vi "Teleop.vi"(10 "Match Info":T4={"Autonomous Elapsed Seconds"=0.0, "TeleOp Elapsed Seconds"=0.0, "Disabled Elapsed Seconds"=0.0, "Visited Autonomous"=FALSE, "Visited TeleOp"=FALSE, "Visited Disabled"=FALSE, "Autonomous Settings"={"Autonomous Style"=enum."Independent", "VI Refnum"=refnum}}, 11 "Call Context":T5) -> ()   [LabVIEW 2016]
doc: "This VI is called for each TeleOp packet received from the DS where the robot is not disabled. It is often used to read from the joysticks and update I/O or to update setpoints for timed control loops. It should complete and return within 20 milliseconds or it may miss DS packets."
uses:
  <vilib>/Rock Robotics/WPI/DriverStation/WPI_DriverStationDerivedRobotMode.ctl
  <vilib>/Rock Robotics/WPI/DriverStation/WPI_DriverStationMatch Info.ctl
  <vilib>/Rock Robotics/WPI/PWM/Servo/WPI_ServoDeviceRef.ctl
  <vilib>/Rock Robotics/SystemInterfaces/DIO/FPGA_DIOPWMChannel.ctl
  <vilib>/Rock Robotics/WPI/PWM/WPI_PWMDeadband.ctl
  <vilib>/Rock Robotics/WPI/Utilities/WPI_GetSetVariantRefNum.vi
  <vilib>/Rock Robotics/Network Tables/NT Write Boolean Array.vi
  <vilib>/Rock Robotics/Network Tables/NT Write Numeric Array.vi
  <vilib>/Rock Robotics/Network Tables/NT Read Boolean.vi
  <vilib>/Rock Robotics/Network Tables/NT Read Number.vi
  <vilib>/Rock Robotics/WPI/RobotDrive/WPI_RobotDriveArcadeDrive_Standard(NoSaturation).vi
  <vilib>/Rock Robotics/WPI/Power/WPI_Power Get 6Volt Rail Voltage and Current.vi
panel:
  in  "x 2":dbl=0.2 format="%#_13g"
  in  "x":dbl=0.2 format="%#_13g"
  out "all currents (A)":dbl[](array[numeric])
  out "current (A)":dbl
  out "all currents (A) 2":dbl[](array[numeric])
  out "PDP current (A)":dbl
  out "PDP voltage (V)":dbl
  out "Power (W)":dbl
  out "Energy (J)":dbl
  out "6 volt rail current (A)":dbl
  out "6 volt rail voltage (V)":dbl
  out "5V User Rail Brown Out":bool
  out "6 V User Rail Short":bool
  out "5 V User Rail Short":bool
  out "3.3V User Rail Short":bool
  out "Input Voltage Brown Out":bool
  out "roboRIO input current (A)":dbl
  out "roboRIO input voltage (V)":dbl
  out "Encoder Status":string
  out "Encoder Rate":dbl
  out "Encoder Direction":string
  out "Encoder Distance":dbl
  out "Gripper Position":dbl
  out "Gripper Servo Device Ref":T1={"DeviceStatus"={"status"=FALSE, "code"=0, "source"=""}, "PWM Channel"=enum."Invalid", "DeadBand"={"Name"="", "maxPositivePwm"=0, "minPositivePwm"=0, "centerPwm"=0, "maxNegativePwm"=0, "minNegativePwm"=0, "angularRange"=0}}
  out "Arm Position":dbl
  out "Arm Servo Device Ref":T1={"DeviceStatus"={"status"=FALSE, "code"=0, "source"=""}, "PWM Channel"=enum."Invalid", "DeadBand"={"Name"="", "maxPositivePwm"=0, "minPositivePwm"=0, "centerPwm"=0, "maxNegativePwm"=0, "minNegativePwm"=0, "angularRange"=0}}
  in  "Gripper Scale Factor":dbl=0.004
  in  "Arm Scale Factor":dbl=0.004
  out "Sample Slider 0":dbl(slide) scale=0.0..5.0
  out "Sample Boolean 1":bool
  out "Sample Boolean 0":bool
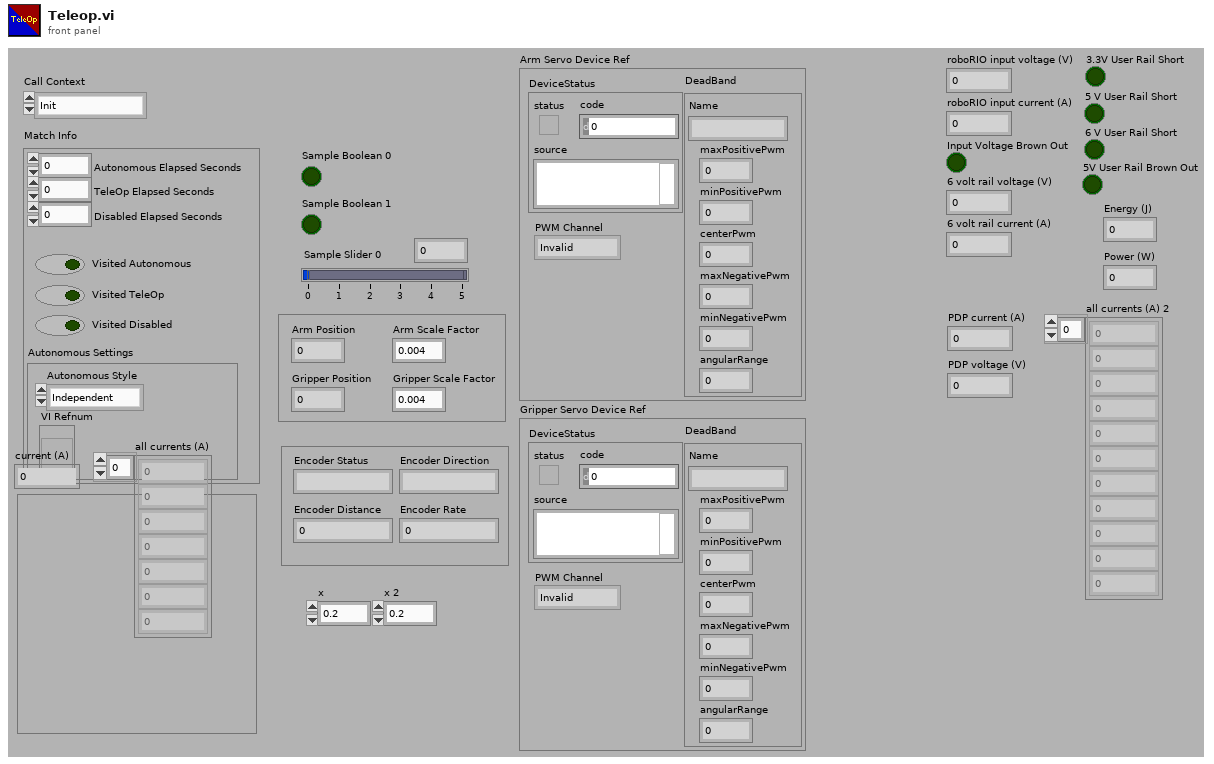
[diagram p1: front panel]
types:
  T1 = typedef "WPI_ServoDeviceRef.ctl" = cluster{"DeviceStatus":errorcluster, "PWM Channel":T2, "DeadBand":T3}
  T2 = typedef "FPGA_DIOPWMChannel.ctl" = enum8{"PWM 0", "PWM 1", "PWM 2", "PWM 3", "PWM 4", "PWM 5", "PWM 6", "PWM 7", "PWM 8", "PWM 9", "PWM MXP 0", "PWM MXP 1", "PWM MXP 2", "PWM MXP 3", "PWM MXP 4", "PWM MXP 5", "PWM MXP 6", "PWM MXP 7", "PWM MXP 8", "PWM MXP 9", "Invalid"}
  T3 = typedef "WPI_PWMDeadband.ctl" = cluster{"Name":string, "maxPositivePwm":i32, "minPositivePwm":i32, "centerPwm":i32, "maxNegativePwm":i32, "minNegativePwm":i32, "angularRange":u16}
  T4 = typedef "WPI_DriverStationMatch Info.ctl" = cluster{"Autonomous Elapsed Seconds":dbl, "TeleOp Elapsed Seconds":dbl, "Disabled Elapsed Seconds":dbl, "Visited Autonomous":bool, "Visited TeleOp":bool, "Visited Disabled":bool, "Autonomous Settings":cluster{"Autonomous Style":enum16{"Iterative", "Independent"}, "VI Refnum":refnum<vi>}}
  T5 = typedef "WPI_DriverStationDerivedRobotMode.ctl" = enum16{"Init", "Execute", "Stop"}
  T6 = typedef "WPI_EncoderDevRef.ctl" = cluster{"DevStatus":errorcluster, "EncoderIndex":T7, "CounterIndex":T8, "DistancePerCount":dbl, "Decoding Type":T9}
  T7 = typedef "FPGA_EncoderIdx.ctl" = enum8{"Enc 0", "Enc 1", "Enc 2", "Enc 3", "Enc 4", "Enc 5", "Enc 6", "Enc 7", "Invalid"}
  T8 = typedef "FPGA_CounterCtrSystemIndex.ctl" = enum8{"Ctr 0", "Ctr 1", "Ctr 2", "Ctr 3", "Ctr 4", "Ctr 5", "Ctr 6", "Ctr 7", "Invalid"}
  T9 = typedef "WPI_EncoderType.ctl" = enum16{"1x", "2x", "4x"}
  T10 = typedef "WPI_RobotDriveDevRef.ctl" = cluster{"DevStatus":errorcluster, "Motors[]":T11[], "Square Inputs":bool, "Max Output":dbl}
  T11 = typedef "WPI_MotorControlDeviceRef.ctl" = cluster{"DeviceStatus":errorcluster, "Type":T12, "PWM":cluster{"PWM Channel":T2, "DeadBand":T3}, "CAN":cluster{"Device Number":u8, "SetOutput VI Ref":variant, "GetOutput VI Ref":variant, "Enable VI Ref":variant, "Disable VI Ref":variant, "Data":variant}, "Invert":bool}
  T12 = typedef "WPI_MotorControlType.ctl" = enum16{"PWM", "CAN"}
  T13 = typedef "WPI_JoystickDevRef.ctl" = cluster{"Device":T14}
  T14 = typedef "WPI_JoystickDeviceEnum.ctl" = enum16{"USB 0", "USB 1", "USB 2", "USB 3", "USB 4", "USB 5"}
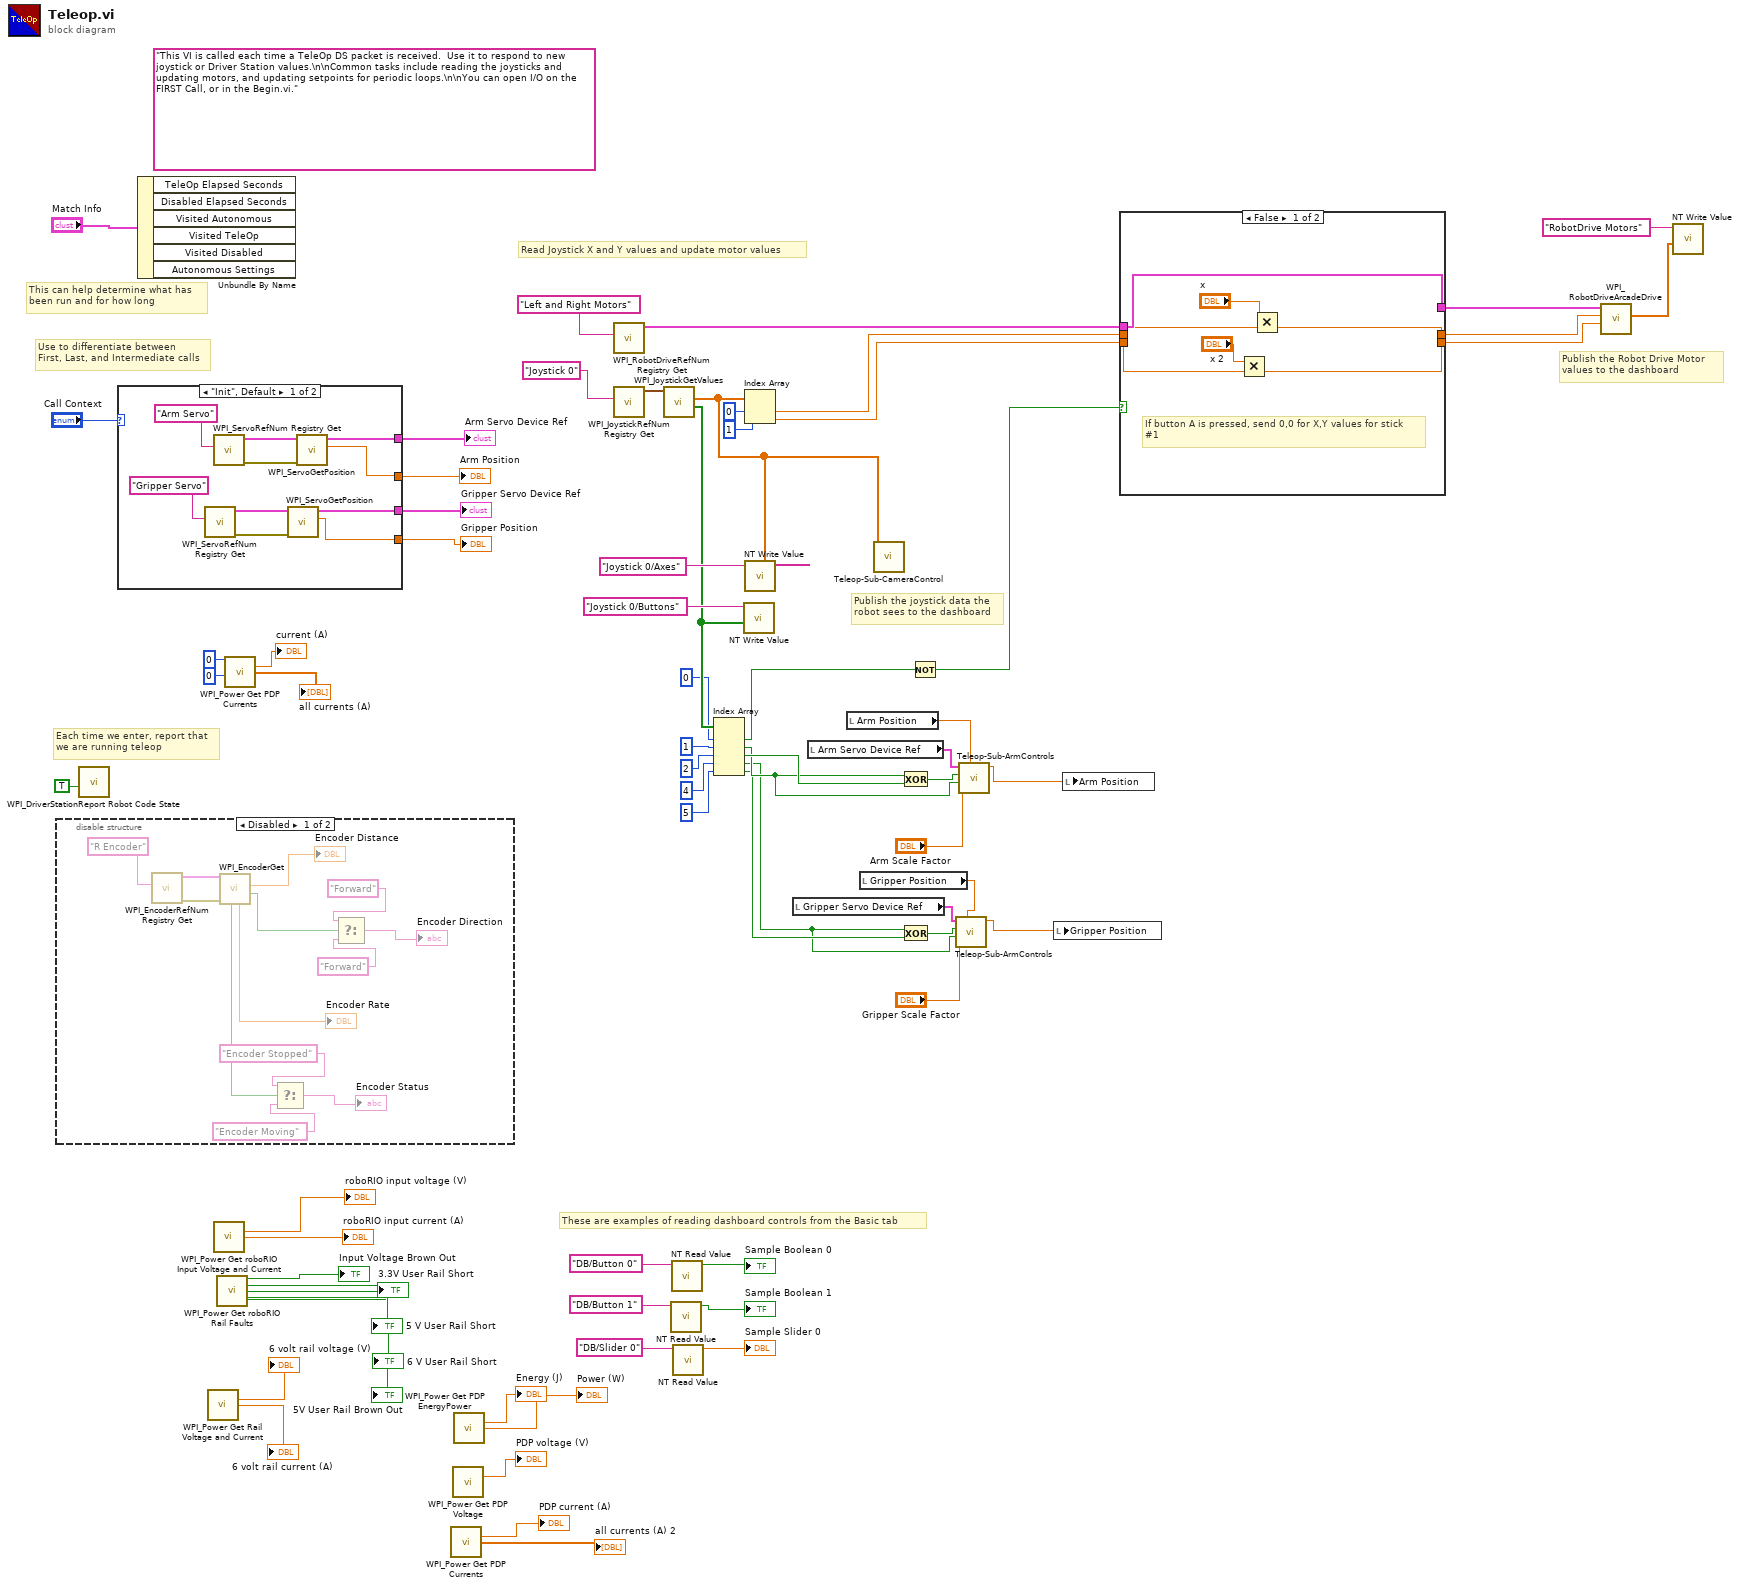
[diagram p0: block diagram]
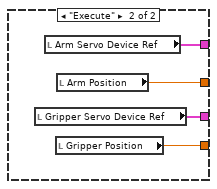
[diagram p3: hidden frame]
diagram:
  (unwired) "This VI is called each time a TeleOp DS packet is received.  Use it to respond to new joystick or Driver Station values.\n\nCommon tasks include reading the joysticks and updating motors, and updating setpoints for periodic loops.\n\nYou can open I/O on the FIRST Call, or in the Begin.vi."
  # "Publish the Robot Drive Motor\nvalues to the dashboard"
  # "These are examples of reading dashboard controls from the Basic tab"
  # "Publish the joystick data the\nrobot sees to the dashboard"
  # "Each time we enter, report that\nwe are running teleop"
  # "Use to differentiate between\nFirst, Last, and Intermediate calls"
  # "This can help determine what has\nbeen run and for how long"
  # "Read Joystick X and Y values and update motor values"
  n1 = disable-structure shown="Disabled" {
    frame Disabled {
      n2 = call <vilib>:"WPI_EncoderRefNum Registry Get.vi"("refnum name"="R Encoder") -> ("error out"=w81:errorcluster, "EncoderDevRef"=w80:T6)  [unwired: 9 in]
      n3 = call <vilib>:"WPI_EncoderGet.vi"("error in (no error)"=w81, "EncoderDevRef"=w80) -> ("Direction"=w78:bool, "Distance"=→"Encoder Distance":dbl, "Rate"=→"Encoder Rate":dbl, "Stopped"=w72:bool)  [unwired: 4 in, 2 out]
      n4 = Select(t="Encoder Stopped" ("refnum name"), s=w72, f="Encoder Moving" ("refnum name")) -> (s? t:f=→"Encoder Status":string)
      n5 = Select(t="Forward" ("refnum name"), s=w78, f="Forward" ("refnum name")) -> (s? t:f=→"Encoder Direction":string)
    }
    frame Enabled {
    }
  }
  n6 = call <vilib>:"WPI_DriverStationReport Robot Code State.vi"("TeleOp"=TRUE ("Autonomous")) -> ()  [unwired: 10 in, 1 out]
  n7 = case shown="\"Init\", Default" "Call Context" {
    tunnel: [w89 w96] -> w30
    tunnel: [w88 w95] -> w29
    tunnel: [w84 w94] -> w28
    tunnel: [w83 w93] -> w25
    frame "Init", Default {
      n8 = call <vilib>:"WPI_ServoRefNum Registry Get.vi"("refnum name"="Gripper Servo") -> ("error out"=w86:errorcluster, "ServoDeviceRef"=w85:T1)  [unwired: 9 in]
      n9 = call <vilib>:"WPI_ServoRefNum Registry Get.vi"("refnum name"="Arm Servo") -> ("error out"=w91:errorcluster, "ServoDeviceRef"=w92:T1)  [unwired: 9 in]
      n10 = call <vilib>:"WPI_ServoGetPosition.vi"("error in (no error)"=w86, "ServoDeviceRef"=w85) -> ("Position"=w83:dbl, "ServoDeviceRef"=w84:T1)  [unwired: 7 in, 1 out]
      n11 = call <vilib>:"WPI_ServoGetPosition.vi"("error in (no error)"=w91, "ServoDeviceRef"=w92) -> ("Position"=w88:dbl, "ServoDeviceRef"=w89:T1)  [unwired: 7 in, 1 out]
    }
    frame "Execute" {
      n12 = local read "Gripper Servo Device Ref"() -> (w94:T1)
      n13 = local read "Arm Servo Device Ref"() -> (w96:T1)
      n14 = local read "Gripper Position"() -> (w93:dbl)
      n15 = local read "Arm Position"() -> (w95:dbl)
    }
  }
  "Arm Servo Device Ref" <- w30
  "Arm Position" <- w29
  "Gripper Servo Device Ref" <- w28
  "Gripper Position" <- w25
  n16 = Unbundle By Name("Match Info") -> ()  [unwired: 6 out]
  n17 = call-poly <vilib>:"WPI_Power Get Rail Voltage and Current.vi"() -> ("6 volt rail voltage (V)"=→"6 volt rail voltage (V)":dbl, "6 volt rail current (A)"=→"6 volt rail current (A)":dbl)  [unwired: 13 in, 1 out]
  n18 = call <vilib>:"WPI_Power Get roboRIO Input Voltage and Current.vi"() -> ("roboRIO input voltage (V)"=→"roboRIO input voltage (V)":dbl, "roboRIO input current (A)"=→"roboRIO input current (A)":dbl)  [unwired: 13 in, 1 out]
  n19 = call <vilib>:"WPI_Power Get roboRIO Rail Faults.vi"() -> ("Input Voltage Brown Out"=→"Input Voltage Brown Out":bool, "3.3V User Rail Short"=→"3.3V User Rail Short":bool, "5 V User Rail Short"=→"5 V User Rail Short":bool, "6 V User Rail Short"=→"6 V User Rail Short":bool, "5V User Rail Brown Out"=→"5V User Rail Brown Out":bool)  [unwired: 10 in, 1 out]
  n20 = call <vilib>:"WPI_Power Get PDP Currents.vi"("Power Distribution Panel (0)"=u8 0, "PDP Channel"=0) -> ("current (A)"=→"current (A)":dbl, "all currents (A)"=→"all currents (A)":dbl[])  [unwired: 11 in, 1 out]
  n21 = call <vilib>:"WPI_Power Get PDP Currents.vi"() -> ("current (A)"=→"PDP current (A)":dbl, "all currents (A)"=→"all currents (A) 2":dbl[])  [unwired: 13 in, 1 out]
  n22 = call <vilib>:"WPI_Power Get PDP Voltage.vi"() -> ("voltage (V)"=→"PDP voltage (V)":dbl)  [unwired: 14 in, 1 out]
  n23 = call <vilib>:"WPI_Power Get PDP EnergyPower.vi"() -> ("Energy (J)"=→"Energy (J)":dbl, "Power (W)"=→"Power (W)":dbl)  [unwired: 13 in, 1 out]
  n24 = call <vilib>:"WPI_RobotDriveRefNum Registry Get.vi"("refnum name"="Left and Right Motors") -> ("RobotDriveDevRef"=w67:T10)  [unwired: 1 in, 9 out]
  n25 = call <vilib>:"WPI_JoystickRefNum Registry Get.vi"("refnum name"="Joystick 0") -> ("JoystickDevRef"=w64:T13)  [unwired: 1 in, 9 out]
  n26 = call <vilib>:"WPI_JoystickGetValues.vi"("JoystickDevRef"=w64) -> ("Buttons"=w47:bool[], "Axes"=w53:dbl[])  [unwired: 6 in, 3 out]
  n27 = call-poly <vilib>:"NT Read Value.vi"("Name"="DB/Button 1" ("refnum name")) -> ("Boolean"=→"Sample Boolean 1":bool)  [unwired: 9 in, 1 out]
  n28 = call-poly <vilib>:"NT Read Value.vi"("Name"="DB/Button 0" ("refnum name")) -> ("Boolean"=→"Sample Boolean 0":bool)  [unwired: 9 in, 1 out]
  n29 = call-poly <vilib>:"NT Read Value.vi"("Name"="DB/Slider 0" ("refnum name")) -> ("Numeric"=→"Sample Slider 0":dbl)  [unwired: 9 in, 1 out]
  n30 = Index Array(array=w47, index #1=0 ("index"), index #2=1 ("index"), index #3=2 ("index"), index #4=4 ("index"), index #5=5 ("index")) -> (element #1=w45:bool, element #2=w37:bool, element #3=w39:bool, element #4=w32:bool, element #5=w33:bool)
  n31 = call-poly <vilib>:"NT Write Value.vi"("Boolean Array"=w47, "Name"="Joystick 0/Buttons") -> ()  [unwired: 9 in, 1 out]
  n32 = Index Array(array=w53, index #1=0 ("index"), index #2=1 ("index")) -> (element #1=w66:dbl, element #2=w62:dbl)
  n33 = call-poly <vilib>:"NT Write Value.vi"("Numeric Array"=w53, "Name"="Joystick 0/Axes") -> ()  [unwired: 9 in, 1 out]
  n34 = local read "Gripper Servo Device Ref"() -> (w23:T1)
  n35 = local read "Arm Servo Device Ref"() -> (w24:T1)
  n36 = local read "Arm Position"() -> (w22:dbl)
  n37 = local read "Gripper Position"() -> (w21:dbl)
  n38 = call "Teleop-Sub-CameraControl.vi"("Axes"=w53) -> ()  [unwired: 11 in]
  n39 = Exclusive Or(1:w39, 2:w37) -> (0:w38:bool)
  n40 = Exclusive Or(1:w33, 2:w32) -> (0:w34:bool)
  n41 = Not(x=w45) -> (.not. x?=w44:bool)
  n42 = call "Teleop-Sub-ArmControls.vi"("ServoDeviceRef"=w23, "Move Arm?"=w34, "Go Up?"=w32, "Scale Factor"="Gripper Scale Factor", "Position In"=w21) -> ("Position"=w26:dbl)  [unwired: 5 in]
  n43 = call "Teleop-Sub-ArmControls.vi"("ServoDeviceRef"=w24, "Move Arm?"=w38, "Go Up?"=w37, "Scale Factor"="Arm Scale Factor", "Position In"=w22) -> ("Position"=w27:dbl)  [unwired: 5 in]
  n44 = local write "Gripper Position"(w26) -> ()
  n45 = local write "Arm Position"(w27) -> ()
  n46 = case shown="False" w44 {
    tunnel: w67 -> [w103 w106]
    tunnel: w66 -> [w102 w105]
    tunnel: w62 -> [w101 w104]
    tunnel: [w103 w106] -> w50
    tunnel: [w98 w105] -> w49
    tunnel: [w100 w104] -> w48
    frame False {
      # "If button A is pressed, send 0,0 for X,Y values for stick\n#1"
      n47 = Multiply(x="x 2", y=w101) -> (x*y=w100:dbl)
      n48 = Multiply(x="x", y=w102) -> (x*y=w98:dbl)
    }
    frame True {
      # "If button is not pressed, pass Axes positions \nthrough."
    }
  }
  n49 = call-poly <vilib>:"WPI_RobotDriveArcadeDrive.vi"("Y axis value"=w48, "X axis value"=w49, "RobotDriveDevRef"=w50) -> ("Motor Values"=w51:dbl[])  [unwired: 6 in, 2 out]
  n50 = call-poly <vilib>:"NT Write Value.vi"("Numeric Array"=w51, "Name"="RobotDrive Motors") -> ()  [unwired: 9 in, 1 out]
